vi "CRYMenu Get Menu Set.vi"(10 "sMenuTag":string) -> (0 "sShortcut_Out":string[](array[string]), 1 "sMultibyte_Out":string[](array[string]), 2 "sID_Out":string[](array[string]), 3 "sUnicode_Out":string[](array[string]))   [LabVIEW 2013]
panel:
  in  "Enable":bool=TRUE
  out "Enable_Out":bool[](array[boolean])
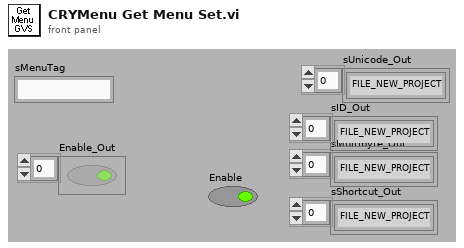
[diagram p1: front panel]
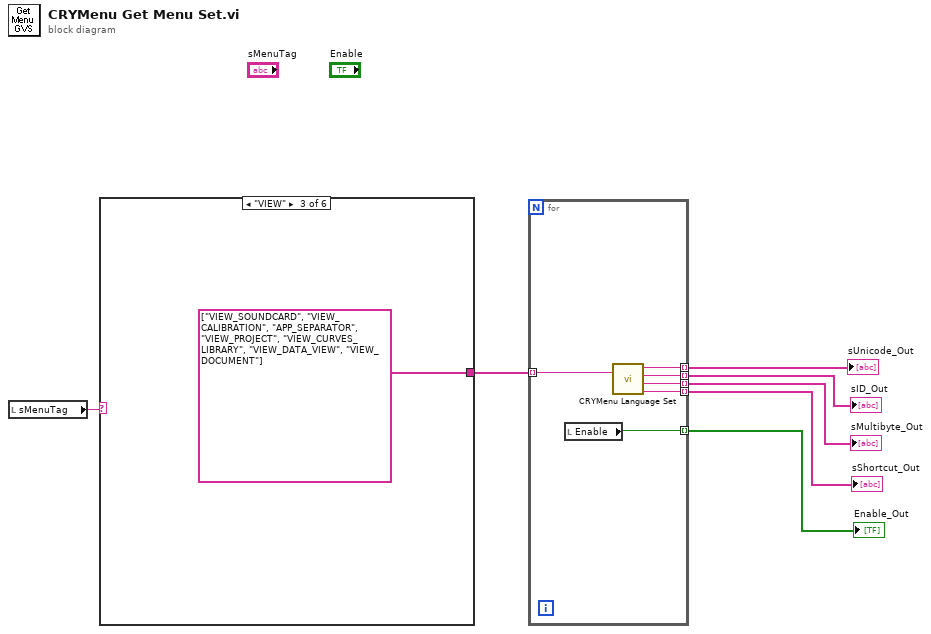
[diagram p0: block diagram]
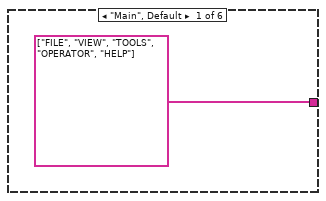
[diagram p2: hidden frame]
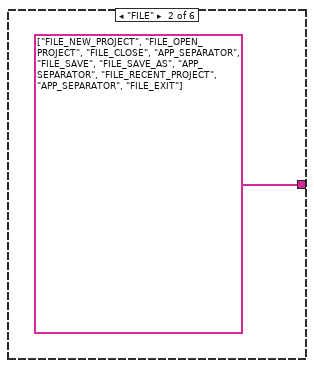
[diagram p3: hidden frame]
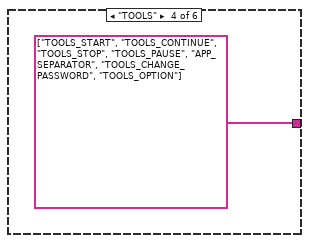
[diagram p4: hidden frame]
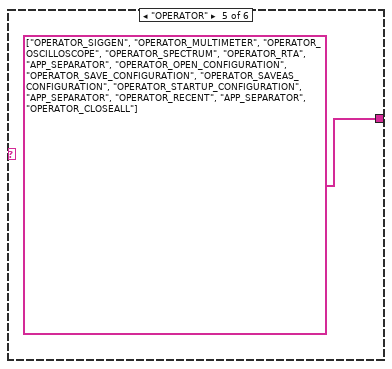
[diagram p5: hidden frame]
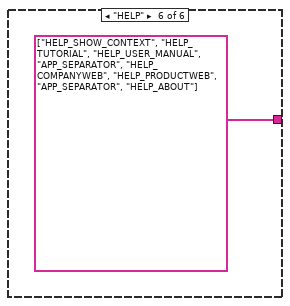
[diagram p6: hidden frame]
diagram:
  n1 = local read "sMenuTag"() -> (w6:string)
  n2 = case shown="\"VIEW\"" w6 {
    tunnel: [string[] ["FILE", "VIEW", "TOOLS", "OPERATOR", "HELP"] string[] ["FILE_NEW_PROJECT", "FILE_OPEN_PROJECT", "FILE_CLOSE", "APP_SEPARATOR", "FILE_SAVE", "FILE_SAVE_AS", "APP_SEPARATOR", "FILE_RECENT_PROJECT", "APP_SEPARATOR", "FILE_EXIT"] string[] ["VIEW_SOUNDCARD", "VIEW_CALIBRATION", "APP_SEPARATOR", "VIEW_PROJECT", "VIEW_CURVES_LIBRARY", "VIEW_DATA_VIEW", "VIEW_DOCUMENT"] string[] ["TOOLS_START", "TOOLS_CONTINUE", "TOOLS_STOP", "TOOLS_PAUSE", "APP_SEPARATOR", "TOOLS_CHANGE_PASSWORD", "TOOLS_OPTION"] string[] ["OPERATOR_SIGGEN", "OPERATOR_MULTIMETER", "OPERATOR_OSCILLOSCOPE", "OPERATOR_SPECTRUM", "OPERATOR_RTA", "APP_SEPARATOR", "OPERATOR_OPEN_CONFIGURATION", "OPERATOR_SAVE_CONFIGURATION", "OPERATOR_SAVEAS_CONFIGURATION", "OPERATOR_STARTUP_CONFIGURATION", "APP_SEPARATOR", "OPERATOR_RECENT", "APP_SEPARATOR", "OPERATOR_CLOSEALL"] string[] ["HELP_SHOW_CONTEXT", "HELP_TUTORIAL", "HELP_USER_MANUAL", "APP_SEPARATOR", "HELP_COMPANYWEB", "HELP_PRODUCTWEB", "APP_SEPARATOR", "HELP_ABOUT"]] -> w7
    frame "Main", Default {
    }
    frame "FILE" {
    }
    frame "VIEW" {
    }
    frame "TOOLS" {
    }
    frame "OPERATOR" {
    }
    frame "HELP" {
    }
  }
  n3 = for {
    tunnel: w7 -> [w19] mode=indexing
    tunnel: [w18] -> w4 mode=indexing
    tunnel: [w17] -> w3 mode=indexing
    tunnel: [w16] -> w2 mode=indexing
    tunnel: [w15] -> w5 mode=indexing
    tunnel: [w14] -> w1 mode=indexing
    n4 = local read "Enable"() -> (w14:bool)
    n5 = call "CRYMenu Language Set.vi"("sID"=w19) -> ("sShortcut_Out"=w16:string, "sMultibyte_Out"=w17:string, "sID_Out"=w18:string, "sUnicode_Out"=w15:string)  [unwired: 7 in]
  }
  "sUnicode_Out" <- w5
  "sMultibyte_Out" <- w3
  "sID_Out" <- w4
  "sShortcut_Out" <- w2
  "Enable_Out" <- w1
